vi "Current VIs Parents Ref__ogtk.vi"() -> (1 "Calling VI's reference":refnum<vi>)   [LabVIEW 2017]
doc: "Gets a reference to the parent of the VI calling this function. This is useful for creating reusable VIs that opperate on their parent."
panel:
  # "[OpenG VI Tags] ***Do Not Remove***"
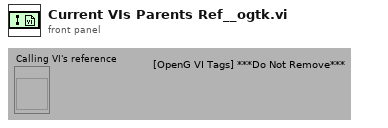
[diagram p1: front panel]
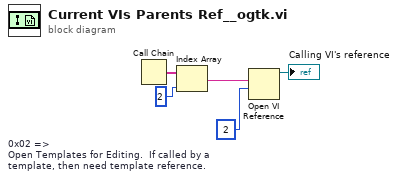
[diagram p0: block diagram]
diagram:
  w1 = 2  # 0x02 => Open Templates for Editing.  If called by a template, then need template reference.
  n1 = Call Chain() -> (call chain=w5:string[])
  n2 = Index Array(array=w5, index=2 ("Index")) -> (element=w3:string)
  n3 = Open VI Reference(vi path=w3, options=w1) -> (vi reference=→"Calling VI's reference":refnum<vi>)  [unwired: 1 in, 4 out]
